vi "Data_get_joe_3.1.vi"() -> ()   [LabVIEW 2011]
uses:
  <vilib>/Utility/error.llb/DialogType.ctl
  <vilib>/Analysis/2dsp.llb/Real FFT.vi
  <vilib>/Analysis/NI_AALPro.lvlib
panel:
  in  "Automatic Overwrite?":bool
  out "f cur. (GHz)":i32
  in  "TDS VISA Port":refnum<visa-resource-name>="GPIB0::1::INSTR"
  in  "Chirp up to (GHz)":dbl
  in  "PauseB":bool caption="Pause"
  in  "Substr":bool
  out "tdsavges#":i32 caption="tds averaged:"
  in  "Auto":bool caption="Autosave"
  in  "FFT every#":u32=1 min=1 max=1000 step=1
  in  "#steps":u32=1 min=1 step=1
  in  "f step (GHz)":dbl=0.0003 min=0.00025 max=67.0 step=1e-06 format="%#.12f"
  in  "time/point":T1(ring)
  in  "time/div":T2(ring)
  out "Current sweep":u32=1 min=1 max=1000 step=1
  in  "Ext":string="ccd"
  in  "Name":string="trace"
  in  "Folder":path
  in  "#Sweeps":u32=1 min=1 max=1000 step=1
  in  "Ampl. (dBm)":dbl min=-135.0 max=30.0 step=0.5 format="%#_8g"
  in  "f start (GHz)":dbl=0.0003 min=0.00025 max=67.0 step=1e-06 format="%#.12f"
  in  "Start":bool
  in  "Quit":bool
  in  "PSG1 VISA Port":refnum<visa-resource-name>="GPIB0::1::INSTR"
  out "read time (ms)":u32
  out "#points":u32
  out "Busy":bool
  in  "Chirp start (MHz)":ext=2.5
  in  "Filter up to (MHz)":ext=2.5
  in  "Amount of averagings":u32=10 min=1 step=1
  out "Data":dbl[](array[numeric])
  out "Frequency Domain Signal":cluster{ext[], dbl[]}(graph)
  out "FFT (Im)":dbl[](array[numeric])
  out "FFT (Re)":dbl[](array[numeric])
  out "Final array":ext[][](array[numeric])
  out "size(s)":i32
  out "Oscilloscope Data":dbl[](array[numeric])
  in  "Channel Number":u16=1
  out "Oscilloscope graph":dbl[](graph)
  in  "Stop":bool
  # "Oscilloscope TDS6124C"
  # "File Storage"
  # "PSG E8257D"
  # "Control"
  # "Spectrum data"
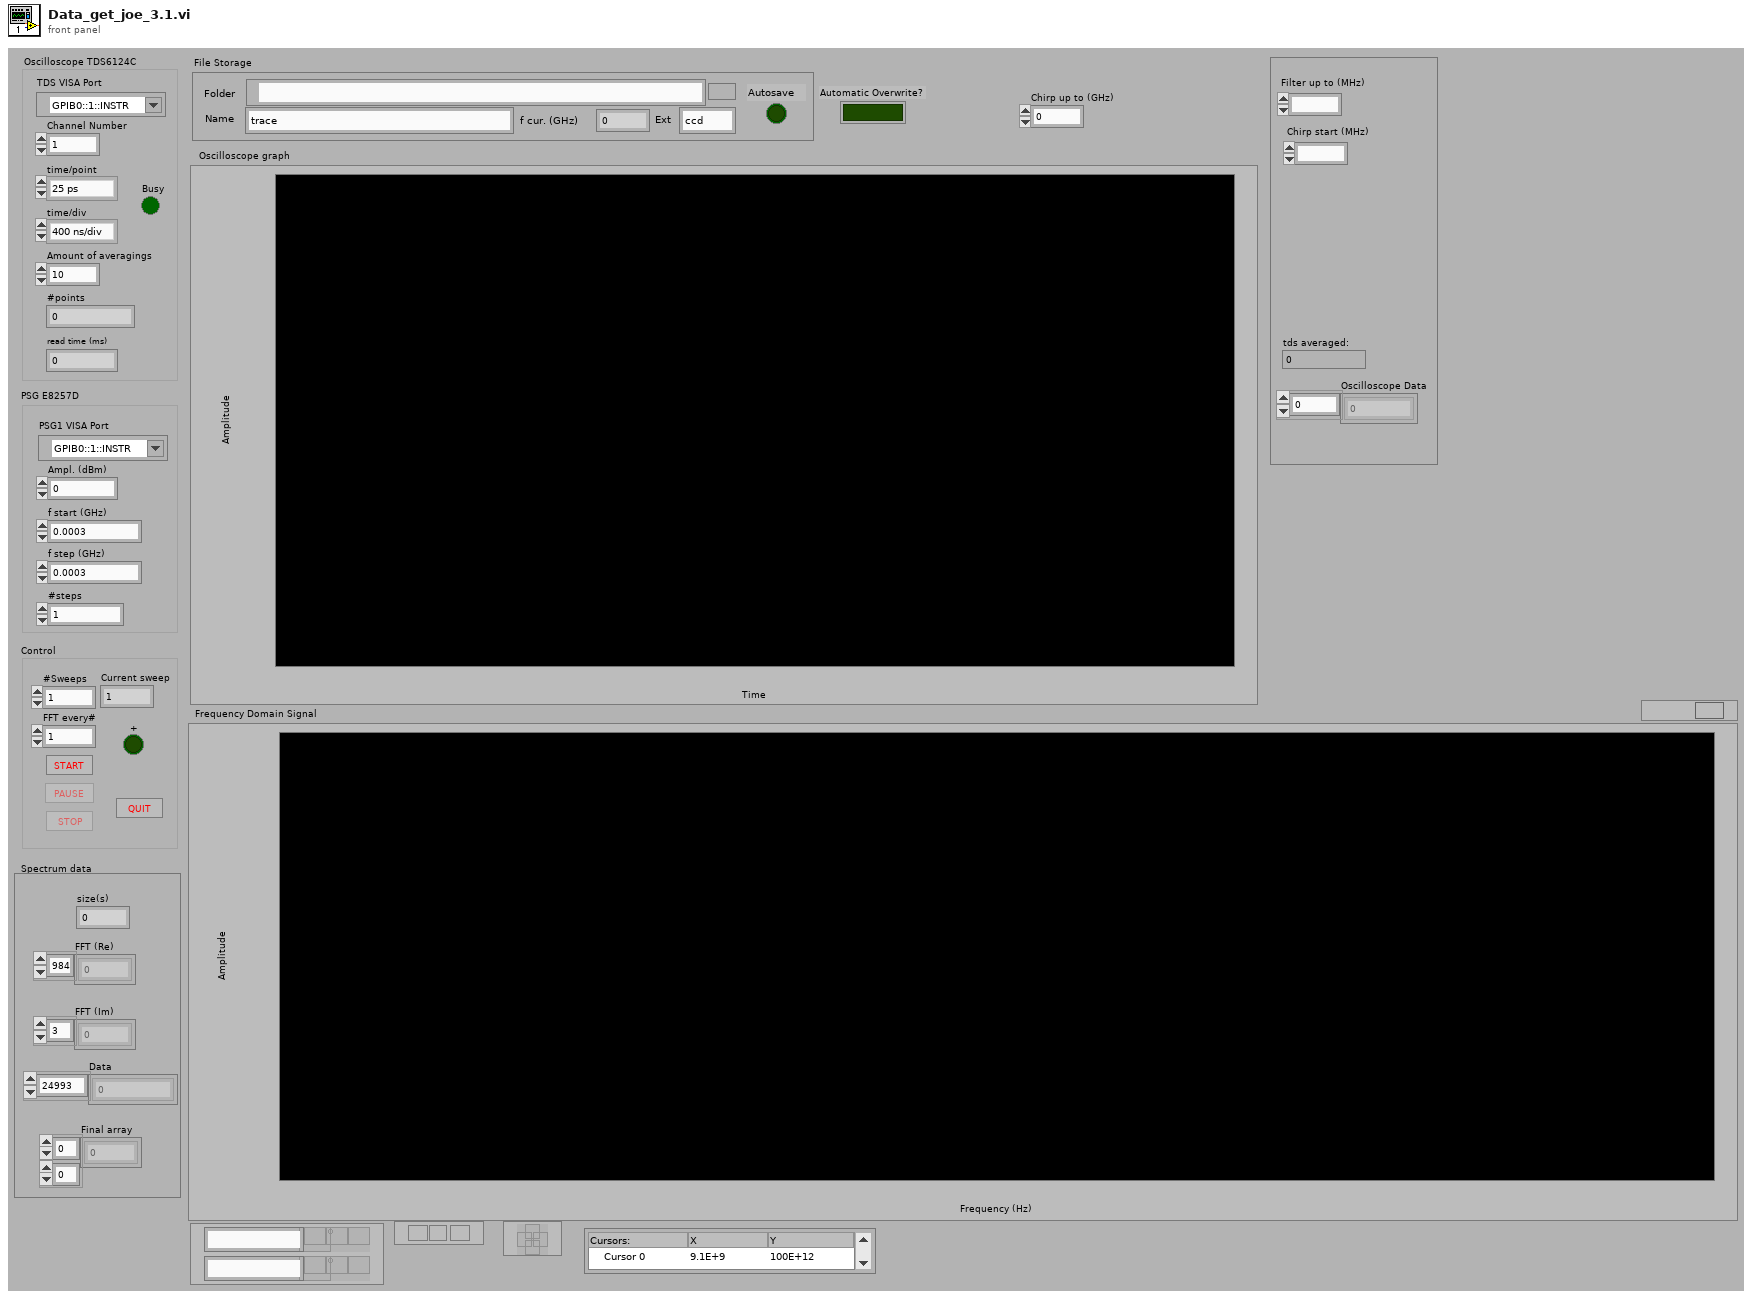
[diagram p1: front panel]
types:
  T1 = enum16{"25 ps", "50 ps", "100 ps", "200 ps", "400 ps", "800 ps", "2 ns"}
  T2 = enum16{"400 ns/div", "1 us/div", "2 us/div", "4 us/div", "10 us/div", "20 us/div"}
  T3 = enum8{"Enabled", "Disabled", "Disabled and Grayed Out"}
  T4 = enum16{"open", "replace", "create", "open or create", "replace or create", "replace or create with confirmation"}
  T5 = typedef "DialogType.ctl" = u16
  T6 = cluster{"Folder":path, "Name":string, "Ext":string}
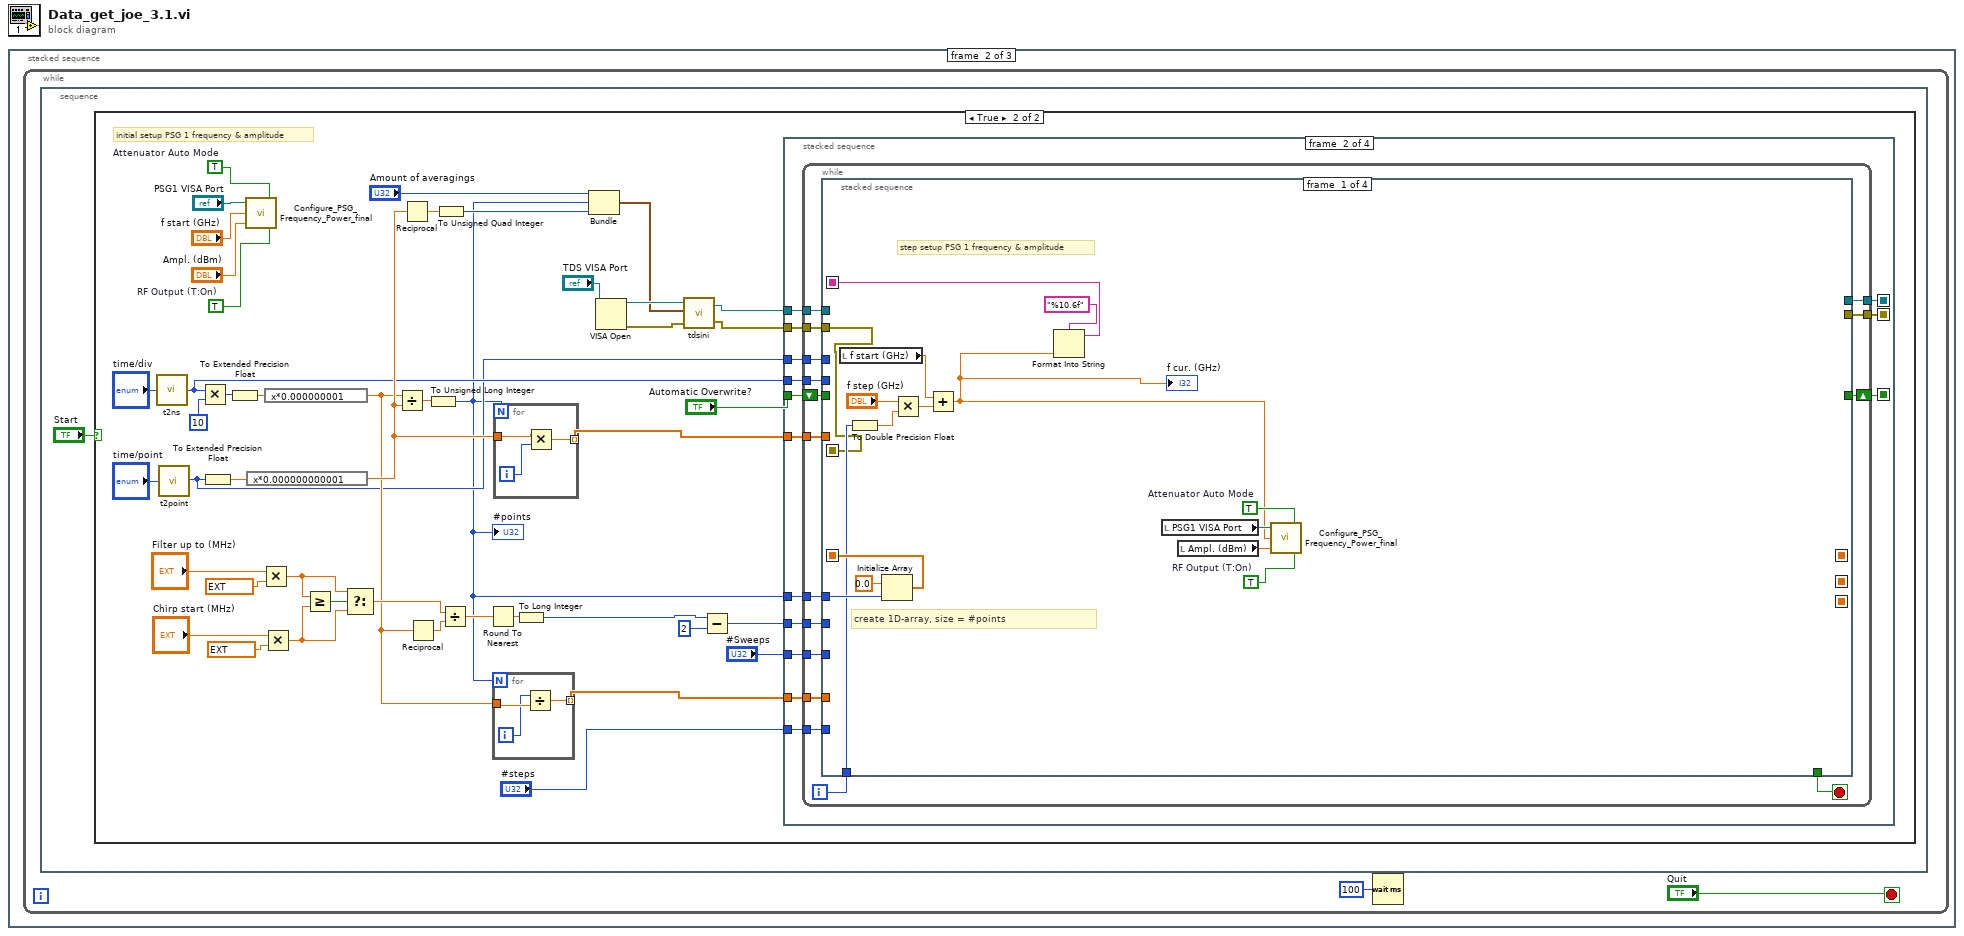
[diagram p0: block diagram]
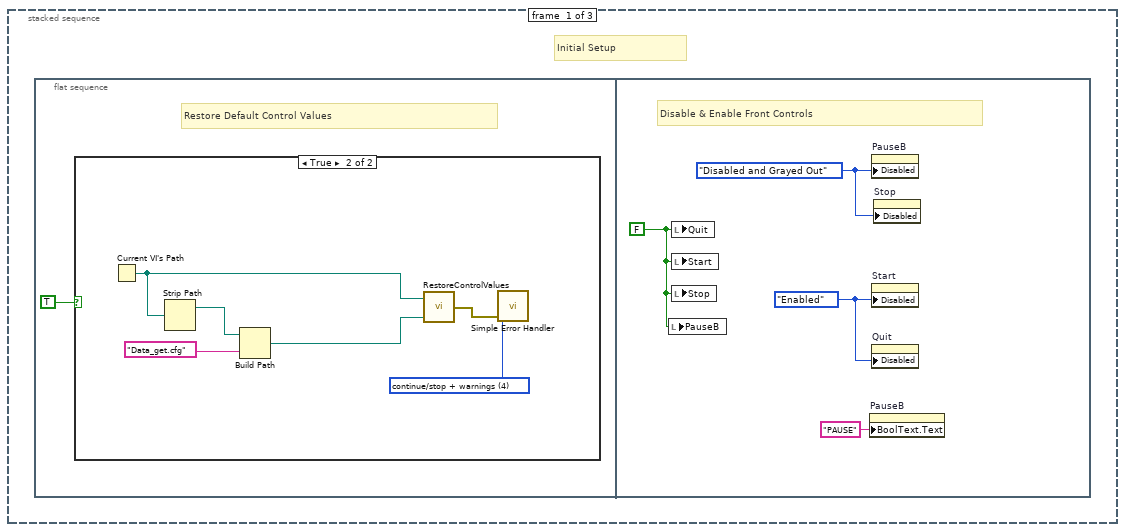
[diagram p2: hidden frame]
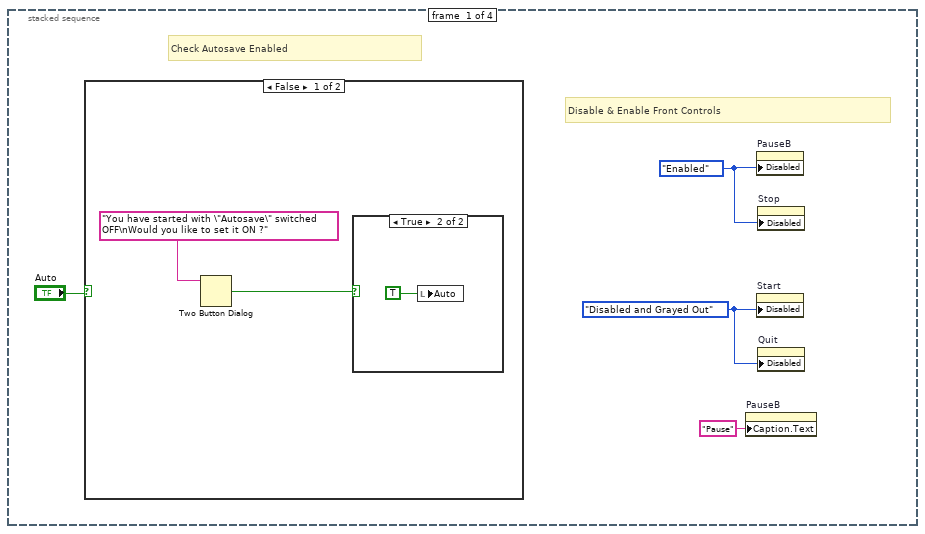
[diagram p5: hidden frame]
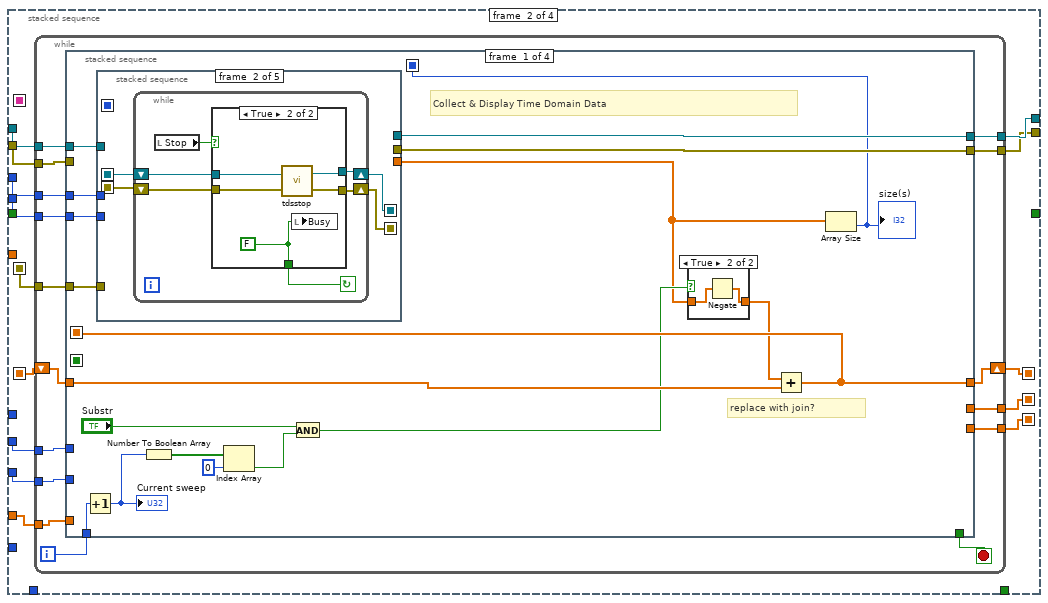
[diagram p8: hidden frame]
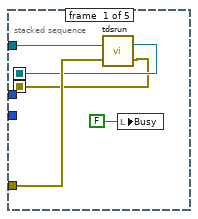
[diagram p10: hidden frame]
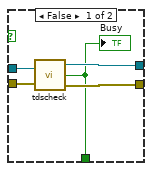
[diagram p11: hidden frame]
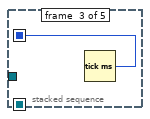
[diagram p12: hidden frame]
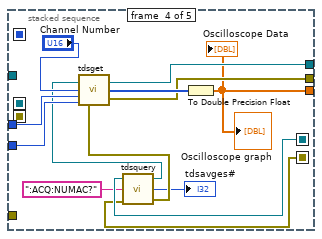
[diagram p13: hidden frame]
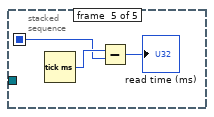
[diagram p14: hidden frame]
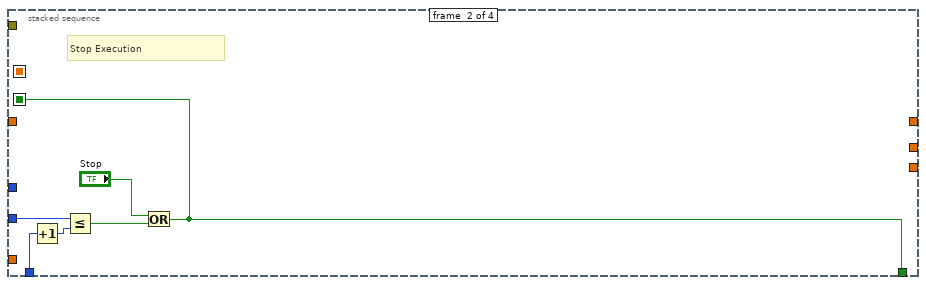
[diagram p15: hidden frame]
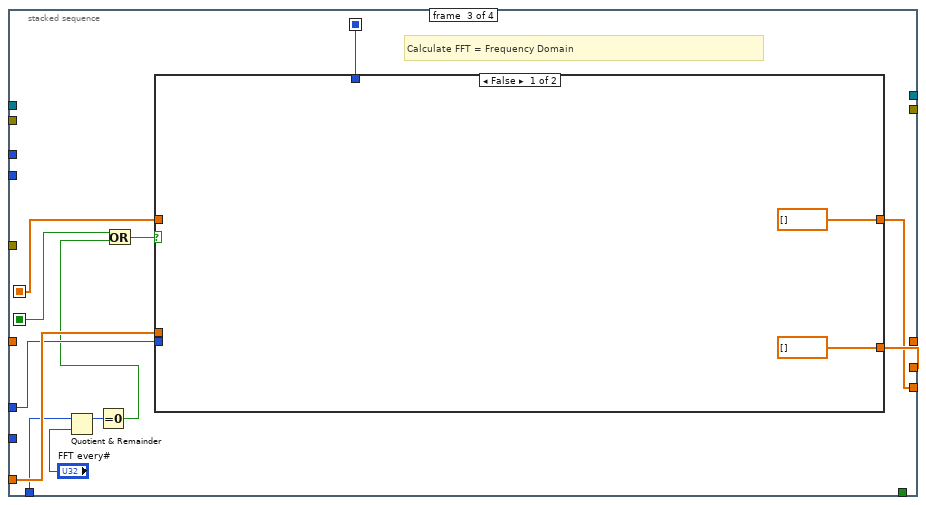
[diagram p16: hidden frame]
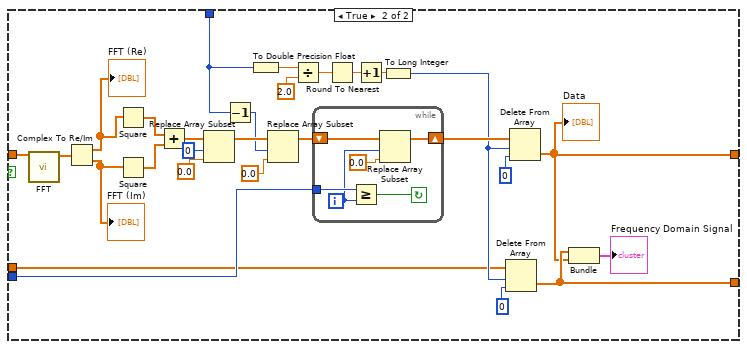
[diagram p17: hidden frame]
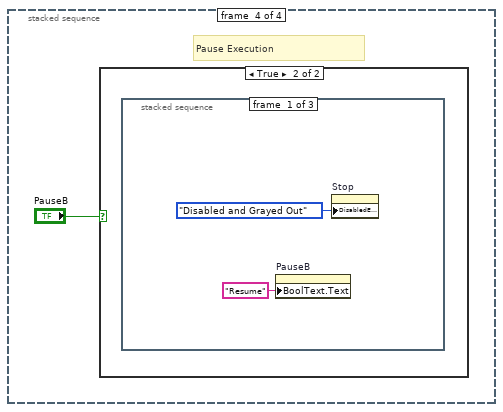
[diagram p18: hidden frame]
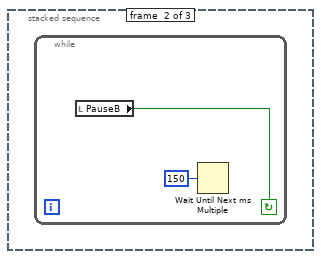
[diagram p20: hidden frame]
diagram:
  n1 = stacked-sequence {
    frame #0 {
      # "Initial Setup"
      n2 = flat-sequence {
        frame #0 {
          # "Restore Default Control Values"
          n3 = case shown="True" TRUE {
            frame False {
            }
            frame True {
              w2 = T5 4 items=["no dialog", "OK message", "continue or stop message", "OK message + warnings", "continue/stop + warnings"] ("type of dialog (OK msg:1)")
              n4 = Current VI's Path() -> (path=w3:path)
              n5 = Strip Path(path=w3) -> (stripped path=w4:path)  [unwired: 1 out]
              n6 = Build Path(base path=w4, name or relative path="Data_get.cfg") -> (appended path=w6:path)
              n7 = call "RestoreControlValues.vi"("file path"=w6, "vi path"=w3) -> ("error out"=w5:errorcluster)
              n8 = call <vilib>:"Simple Error Handler.vi"("type of dialog (OK msg:1)"=w2, "error in (no error)"=w5) -> ()  [unwired: 3 in, 5 out]
            }
          }
        }
        frame #1 {
          w10 = T3."Disabled and Grayed Out" ("Disabled")
          w8 = T3."Enabled" ("Disabled")
          w11 = FALSE ("Quit")
          # "Disable & Enable Front Controls"
          n9 = local write "PauseB"(w11) -> ()
          n10 = local write "Quit"(w11) -> ()
          n11 = local write "Start"(w11) -> ()
          n12 = local write "Stop"(w11) -> ()
          n13 = property on="PauseB" class="Bool (strict)"("BoolText.Text"="PAUSE" ("Boolean Text.Text")) -> ()  [unwired: 2 in, 2 out]
          n14 = property on="PauseB" class="Bool (strict)"("Disabled"=w10) -> ()  [unwired: 2 in, 2 out]
          n15 = property on="Start" class="Bool (strict)"("Disabled"=w8) -> ()  [unwired: 2 in, 2 out]
          n16 = property on="Quit" class="Bool (strict)"("Disabled"=w8) -> ()  [unwired: 2 in, 2 out]
          n17 = property on="Stop" class="Bool (strict)"("Disabled"=w10) -> ()  [unwired: 2 in, 2 out]
        }
      }
    }
    frame #1 {
      n18 = while {
        stop <- "Quit" stop-if-true
        n19 = stacked-sequence {
          frame #0 {
            n20 = case shown="True" "Start" {
              frame False {
              }
              frame True {
                w19 = TRUE  # Attenuator Auto Mode
                w16 = TRUE  # RF Output (T:On)
                # "initial setup PSG 1 frequency & amplitude"
                n21 = call "t2ns.vi"("t/div"="time/div") -> ("ns/div"=w31:u32)
                n22 = call "t2point.vi"("t/point"="time/point") -> ("ps/point"=w29:u32)
                n23 = Multiply(x=w31, y=u32 10) -> (x*y=w54:u32)
                n24 = To Extended Precision Float(1:w29) -> (0:w51:ext)
                n25 = To Extended Precision Float(1:w54) -> (0:w52:ext)
                n26 = call "Configure_PSG_ Frequency_Power_final.vi"("RF Output (T:On)"=w16, "Attenuator Auto Mode (T:Enable)"=w19, "Power [dBm]"="Ampl. (dBm)", "Frequency [GHz]"="f start (GHz)", "VISA resource name"="PSG1 VISA Port") -> ()
                n27 = expression code="x*0.000000000001"(w51) -> (w37:ext)
                n28 = Multiply(x="Filter up to (MHz)", y=ext 1000000.0) -> (x*y=w43:ext)
                n29 = Multiply(x="Chirp start (MHz)", y=ext 1000000.0) -> (x*y=w40:ext)
                n30 = expression code="x*0.000000001"(w52) -> (w33:ext)
                n31 = Greater Or Equal?(x=w43, y=w40) -> (x >= y?=w50:bool)
                n32 = Select(t=w43, s=w50, f=w40) -> (s? t:f=w48:ext)
                n33 = Divide(x=w33, y=w37) -> (x/y=w53:ext)
                n34 = Reciprocal(x=w37) -> (1/x=w35:ext)
                n35 = Reciprocal(x=w33) -> (1/x=w49:ext)
                n36 = To Unsigned Long Integer(number=w53) -> (unsigned 32bit integer=w27:u32)
                "#points" <- w27
                n37 = To Unsigned Quad Integer(1:w35) -> (0:w36:u64)
                n38 = Divide(x=w48, y=w49) -> (x/y=w47:ext)
                n39 = Round To Nearest(number=w47) -> (nearest integer value=w46:ext)
                n40 = for {
                  N: w27 -> [_]
                  tunnel: w33 -> [w458]
                  tunnel: [w459] -> w34 mode=indexing
                  i -> [w457]
                  n41 = Divide(x=w457, y=w458) -> (x/y=w459:ext)
                }
                n42 = for {
                  N: w27 -> [_]
                  tunnel: w37 -> [w462]
                  tunnel: [w461] -> w32 mode=indexing
                  i -> [w460]
                  n43 = Multiply(x=w462, y=w460) -> (x*y=w461:ext)
                }
                n44 = To Long Integer(number=w46) -> (32bit integer=w24:i32)
                n45 = Bundle("Amount of averagings"="Amount of averagings", w27, w36) -> (w38:cluster{"Amount of averagings ":u32, u32, u64})  [unwired: 1 in]
                n46 = VISA Open(VISA resource name="TDS VISA Port") -> (VISA resource name=w56:refnum<visa-resource-name>, error out=w57:errorcluster)  [unwired: 4 in]
                n47 = call "tdsini.vi"("Error In (No Error)"=w57, "Acq_par"=w38, "VISA Port In"=w56) -> ("Error Out"=w58:errorcluster, "VISA Port Out"=w59:refnum<visa-resource-name>)
                n48 = Subtract(x=w24, y=2) -> (x-y=w22:i32)
                n49 = stacked-sequence {
                  seq-local: [_ w73 _ _] -> [_ _ w418 _]
                  seq-local: [_ w72 _ _] -> [_ _ w417 _]
                  seq-local: [_ w67 _ _] -> [_ _ _ w419]
                  tunnel: w59 -> [_ w80 _ _]
                  tunnel: w58 -> [_ w79 _ _]
                  tunnel: w29 -> [_ w78 _ _]
                  tunnel: w31 -> [_ w77 _ _]
                  tunnel: w22 -> [_ w76 _ _]
                  tunnel: w34 -> [_ w75 _ _]
                  tunnel: "#Sweeps" -> [_ w74 _ _]
                  tunnel: w32 -> [_ w69 _ _]
                  tunnel: w27 -> [_ w71 _ _]
                  tunnel: "#steps" -> [_ w70 _ _]
                  tunnel: "Automatic Overwrite?" -> [_ w68 _ _]
                  frame #0 {
                    w61 = T3."Enabled" ("Disabled")
                    w60 = T3."Disabled and Grayed Out" ("Disabled")
                    # "Check Autosave Enabled"
                    # "Disable & Enable Front Controls"
                    n50 = case shown="False" "Auto" {
                      frame False {
                        n51 = Two Button Dialog(message="You have started with \"Autosave\" switched OFF\nWould you like to set it ON ?") -> (T button?=w64:bool)  [unwired: 2 in]
                        n52 = case shown="True" w64 {
                          frame False {
                          }
                          frame True {
                            n53 = local write "Auto"(TRUE) -> ()
                          }
                        }
                      }
                      frame True {
                      }
                    }
                    n54 = property on="PauseB" class="Bool (strict)"("Caption.Text"="Pause") -> ()  [unwired: 2 in, 2 out]
                    n55 = property on="PauseB" class="Bool (strict)"("Disabled"=w61) -> ()  [unwired: 2 in, 2 out]
                    n56 = property on="Start" class="Bool (strict)"("Disabled"=w60) -> ()  [unwired: 2 in, 2 out]
                    n57 = property on="Stop" class="Bool (strict)"("Disabled"=w61) -> ()  [unwired: 2 in, 2 out]
                    n58 = property on="Quit" class="Bool (strict)"("Disabled"=w60) -> ()  [unwired: 2 in, 2 out]
                  }
                  frame #1 {
                    n59 = while {
                      tunnel: w80 -> [w96]
                      tunnel: w79 -> [w95]
                      tunnel: w78 -> [w94]
                      tunnel: w77 -> [w93]
                      tunnel: w76 -> [w92]
                      tunnel: w75 -> [w91]
                      tunnel: w74 -> [w90]
                      tunnel: [w89] -> w73
                      tunnel: [w88] -> w72
                      tunnel: w71 -> [w87]
                      tunnel: w70 -> [w85]
                      tunnel: w69 -> [w83]
                      shift-right: [w81] -> w67
                      shift-left: w68 -> [w82]
                      i -> [w86]
                      stop <- w84 stop-if-true
                      n60 = stacked-sequence {
                        seq-local: [w111 _ _ _] -> [_ w117 _ _]
                        seq-local: [w102 _ _ _] -> [_ w116 _ _]
                        seq-local: [_ w115 _ _] -> [_ _ w273 _]
                        seq-local: [_ w114 _ _] -> [_ _ w272 _]
                        seq-local: [_ w113 _ _] -> [_ _ w271 _]
                        seq-local: [w103 _ _ _] -> [_ _ w270 _]
                        tunnel: w96 -> [_ w126 _ _]
                        tunnel: w95 -> [w102 w125 _ _]
                        tunnel: w94 -> [_ w124 _ _]
                        tunnel: w93 -> [_ w123 _ _]
                        tunnel: w92 -> [_ w122 _ _]
                        tunnel: w91 -> [_ w121 _ _]
                        tunnel: w90 -> [_ w120 _ _]
                        tunnel: [_ w119 _ _] -> w89
                        tunnel: [_ w118 _ _] -> w88
                        tunnel: w87 -> [w110 _ _ _]
                        tunnel: w86 -> [w107 _ _ w411]
                        tunnel: w85 -> [_ _ _ w410]
                        tunnel: [_ _ _ w409] -> w84
                        tunnel: w83 -> [_ _ w274 _]
                        tunnel: w82 -> [_ _ w268 _]
                        tunnel: [_ _ w267 _] -> w81
                        frame #0 {
                          w101 = TRUE  # Attenuator Auto Mode
                          w100 = TRUE  # RF Output (T:On)
                          # "step setup PSG 1 frequency & amplitude"
                          # "create 1D-array, size = #points"
                          n61 = local read "f start (GHz)"() -> (w105:dbl)
                          n62 = To Double Precision Float(number=w107) -> (double precision float=w108:dbl)
                          n63 = Initialize Array(0.0 ("element"), w110) -> (w111:dbl[])
                          n64 = Multiply(x="f step (GHz)", y=w108) -> (x*y=w106:dbl)
                          n65 = Add(x=w105, y=w106) -> (x+y=w98:dbl)
                          "f cur. (GHz)" <- w98
                          n66 = Format Into String(format string="%10.6f", w98) -> (resulting string=w103:string)  [unwired: 2 in, 1 out]
                          n67 = local read "PSG1 VISA Port"() -> (w99:refnum<visa-resource-name>)
                          n68 = local read "Ampl. (dBm)"() -> (w97:dbl)
                          n69 = call "Configure_PSG_ Frequency_Power_final.vi"("RF Output (T:On)"=w100, "Attenuator Auto Mode (T:Enable)"=w101, "Power [dBm]"=w97, "Frequency [GHz]"=w98, "VISA resource name"=w99) -> ()
                        }
                        frame #1 {
                          n70 = while {
                            tunnel: [w139] -> w118
                            tunnel: [w140] -> w119
                            tunnel: w125 -> [w141]
                            tunnel: w126 -> [w142]
                            tunnel: w124 -> [w138]
                            tunnel: w123 -> [w137]
                            tunnel: w121 -> [w135]
                            tunnel: w122 -> [w136]
                            tunnel: w120 -> [w132]
                            shift-right: [w130] -> w115
                            shift-left: w117 -> [w131]
                            tunnel: [w129] -> w114
                            tunnel: w116 -> [w128]
                            tunnel: [w127] -> w113
                            i -> [w134]
                            stop <- w133 stop-if-true
                            n71 = stacked-sequence {
                              seq-local: [w152 _ _ _] -> [_ _ w223 _]
                              seq-local: [w153 _ _ _] -> [_ _ w222 _]
                              seq-local: [_ w206 _ _] -> [_ _ w213 _]
                              tunnel: w142 -> [w160 _ _ _]
                              tunnel: w141 -> [_ _ _ _]
                              tunnel: [w159 _ _ _] -> w140
                              tunnel: [w158 _ _ _] -> w139
                              tunnel: w138 -> [w157 _ _ _]
                              tunnel: w137 -> [w156 _ _ _]
                              tunnel: w136 -> [_ _ w220 _]
                              tunnel: w135 -> [_ _ w221 _]
                              tunnel: w134 -> [w151 w211 w217 _]
                              tunnel: [_ w206 _ _] -> w133
                              tunnel: w132 -> [_ w208 _ _]
                              tunnel: w131 -> [w155 _ _ _]
                              tunnel: [w153 _ _ _] -> w130
                              tunnel: [_ _ w219 _] -> w129
                              tunnel: w128 -> [w154 _ _ _]
                              tunnel: [_ _ w218 _] -> w127
                              frame #0 {
                                # "replace with join?"
                                # "Collect & Display Time Domain Data"
                                n72 = Increment(x=w151) -> (x+1=w143:i32)
                                "Current sweep" <- w143
                                n73 = stacked-sequence {
                                seq-local: [w166 _ _ _ _] -> [_ w172 _ _ _]
                                seq-local: [w165 _ _ _ _] -> [_ w171 _ _ _]
                                seq-local: [_ w169 _ _ _] -> [_ _ _ w194 _]
                                seq-local: [_ w170 _ _ _] -> [_ _ _ w195 _]
                                seq-local: [_ _ w189 _ _] -> [_ _ _ _ w204]
                                tunnel: w160 -> [w167 _ _ _ _]
                                tunnel: w154 -> [w168 _ _ _ _]
                                tunnel: [_ _ _ w201 _] -> w159
                                tunnel: [_ _ _ w200 _] -> w158
                                tunnel: w157 -> [_ _ _ w198 _]
                                tunnel: w156 -> [_ _ _ w197 _]
                                tunnel: [_ _ _ w196 _] -> w146
                                frame #0 {
                                n74 = call "tdsrun.vi"("Error In (No Error)"=w168, "VISA Port In"=w167) -> ("Error Out"=w165:errorcluster, "VISA Port Out"=w166:refnum<visa-resource-name>)
                                n75 = local write "Busy"(FALSE ("Busy")) -> ()
                                }
                                frame #1 {
                                n76 = while {
                                shift-right: [w176] -> w170
                                shift-left: w172 -> [w177]
                                shift-right: [w175] -> w169
                                shift-left: w171 -> [w178]
                                stop <- w174 continue-if-true
                                n77 = local read "Stop"() -> (w173:bool)
                                n78 = case shown="True" w173 {
                                tunnel: w178 -> [w183 w187]
                                tunnel: w177 -> [w182 w188]
                                tunnel: [w181 w185] -> w176
                                tunnel: [w180 w186] -> w175
                                tunnel: [w179 w184] -> w174
                                frame False {
                                n79 = call "tdscheck.vi"("VISA Port In"=w182, "Error In (No Error)"=w183) -> ("VISA Port Out"=w181:refnum<visa-resource-name>, "busy"=w179:bool, "Error Out"=w180:errorcluster)
                                "Busy" <- w179
                                }
                                frame True {
                                w184 = FALSE ("busy")
                                n80 = call "tdsstop.vi"("Error In (No Error)"=w187, "VISA Port In"=w188) -> ("Error Out"=w186:errorcluster, "VISA Port Out"=w185:refnum<visa-resource-name>)
                                n81 = local write "Busy"(w184) -> ()
                                }
                                }
                                }
                                }
                                frame #2 {
                                n82 = Tick Count (ms)() -> (millisecond timer value=w189:u32)
                                }
                                frame #3 {
                                n83 = call "tdsquery.vi"("Error In (No Error)"=w194, "String to TDS"=":ACQ:NUMAC?", "VISA Port In"=w195) -> ("Error Out"=w191:errorcluster, "number"=→"tdsavges#":i32, "VISA Port Out"=w192:refnum<visa-resource-name>)
                                n84 = call "tdsget.vi"("VISA Port In"=w192, "Channel Number"="Channel Number", "ps/point"=w198, "ns/div"=w197, "Error In (No Error)"=w191) -> ("VISA Port Out"=w201:refnum<visa-resource-name>, "TDS Data"=w202:u16[], "Error Out"=w200:errorcluster)  [unwired: 8 in]
                                n85 = To Double Precision Float(number=w202) -> (double precision float=w196:dbl[])
                                "Oscilloscope graph" <- w196
                                "Oscilloscope Data" <- w196
                                }
                                frame #4 {
                                n86 = Tick Count (ms)() -> (millisecond timer value=w205:u32)
                                n87 = Subtract(x=w205, y=w204) -> (x-y=→"read time (ms)":u32)
                                }
                                }
                                n88 = Number To Boolean Array(number=w143) -> (Boolean array=w150:bool[])
                                n89 = Index Array(array=w150, index=0) -> (element=w148:bool)
                                n90 = And(x="Substr", y=w148) -> (x .and. y?=w147:bool)
                                n91 = case shown="True" w147 {
                                tunnel: w146 -> [w161 w163]
                                tunnel: [w161 w162] -> w145
                                frame False {
                                }
                                frame True {
                                n92 = Negate(x=w163) -> (-x=w162:dbl[])
                                }
                                }
                                n93 = Add(x=w145, y=w155) -> (x+y=w153:dbl[])
                                n94 = Array Size(array=w146) -> (size(s)=w152:i32)
                                "size(s)" <- w152
                              }
                              frame #1 {
                                # "Stop Execution"
                                n95 = Increment(x=w211) -> (x+1=w207:i32)
                                n96 = Less Or Equal?(x=w208, y=w207) -> (x <= y?=w210:bool)
                                n97 = Or(x="Stop", y=w210) -> (x .or. y?=w206:bool)
                              }
                              frame #2 {
                                # "Calculate FFT = Frequency Domain"
                                n98 = Quotient & Remainder(x=w217, y="FFT every#") -> (x-y*floor(x/y)=w215:u32)  [unwired: 1 out]
                                n99 = Equal To 0?(x=w215) -> (x = 0?=w212:bool)
                                n100 = Or(x=w213, y=w212) -> (x .or. y?=w214:bool)
                                n101 = case shown="False" w214 {
                                tunnel: w223 -> [_ w231]
                                tunnel: w222 -> [_ w230]
                                tunnel: w221 -> [_ w226]
                                tunnel: w220 -> [_ w229]
                                tunnel: [ext[] [] w228] -> w219
                                tunnel: [dbl[] [] w227] -> w218
                                frame False {
                                }
                                frame True {
                                n102 = call-poly <vilib>:"FFT.vi"("X"=w230) -> ("FFT {X}"=w253:cdb[])  [unwired: 9 in, 1 out]
                                n103 = Complex To Re/Im(x + iy=w253) -> (x=w252:dbl[], y=w251:dbl[])
                                "FFT (Re)" <- w252
                                "FFT (Im)" <- w251
                                n104 = Square(x=w252) -> (x^2=w250:dbl[])
                                n105 = Square(x=w251) -> (x^2=w249:dbl[])
                                n106 = Add(x=w250, y=w249) -> (x+y=w245:dbl[])
                                n107 = Replace Array Subset(array=w245, new element=0.0 ("new element/subarray"), index=0) -> (w244:dbl[])
                                n108 = Decrement(x=w231) -> (x-1=w243:i32)
                                n109 = To Double Precision Float(number=w231) -> (double precision float=w239:dbl)
                                n110 = Replace Array Subset(array=w244, new element=0.0 ("new element/subarray"), index=w243) -> (w241:dbl[])
                                n111 = Divide(x=w239, y=2.0) -> (x/y=w237:dbl)
                                n112 = while {
                                tunnel: w229 -> [w258]
                                shift-right: [w256] -> w240
                                shift-left: w241 -> [w257]
                                i -> [w255]
                                stop <- w259 continue-if-true
                                n113 = Greater Or Equal?(x=w258, y=w255) -> (x >= y?=w259:bool)
                                n114 = Replace Array Subset(array=w257, new element=0.0 ("new element/subarray"), index=w255) -> (w256:dbl[])
                                }
                                n115 = Round To Nearest(number=w237) -> (nearest integer value=w236:dbl)
                                n116 = Increment(x=w236) -> (x+1=w235:dbl)
                                n117 = To Long Integer(number=w235) -> (32bit integer=w232:i32)
                                n118 = Delete From Array(array=w226, length=w232, index=0) -> (deleted portion=w228:ext[])  [unwired: 1 out]
                                n119 = Delete From Array(array=w240, length=w232, index=0) -> (deleted portion=w227:dbl[])  [unwired: 1 out]
                                "Data" <- w227
                                n120 = Bundle(w228, w227) -> (→"Frequency Domain Signal":cluster{ext[], dbl[]})  [unwired: 1 in]
                                }
                                }
                              }
                              frame #3 {
                                # "Pause Execution"
                                n121 = case shown="True" "PauseB" {
                                frame False {
                                }
                                frame True {
                                n122 = stacked-sequence {
                                frame #0 {
                                n123 = property on="PauseB" class="Bool (strict)"("BoolText.Text"="Resume" ("Caption.Text")) -> ()  [unwired: 2 in, 2 out]
                                n124 = property on="Stop" class="Bool (strict)"("DisabledEnum"=T3."Disabled and Grayed Out" ("Disabled")) -> ()  [unwired: 2 in, 2 out]
                                }
                                frame #1 {
                                n125 = while {
                                stop <- w264 continue-if-true
                                n126 = local read "PauseB"() -> (w264:bool)
                                n127 = Wait Until Next ms Multiple(millisecond multiple=u32 150) -> ()  [unwired: 1 out]
                                }
                                }
                                frame #2 {
                                n128 = property on="PauseB" class="Bool (strict)"("BoolText.Text"="Pause" ("Caption.Text")) -> ()  [unwired: 2 in, 2 out]
                                n129 = property on="Stop" class="Bool (strict)"("DisabledEnum"=T3."Enabled" ("Disabled")) -> ()  [unwired: 2 in, 2 out]
                                }
                                }
                                }
                                }
                              }
                            }
                          }
                        }
                        frame #2 {
                          # "Auto Safe?"
                          n130 = local read "Auto"() -> (w269:bool)
                          n131 = case shown="True" w269 {
                            tunnel: w274 -> [_ w282]
                            tunnel: w273 -> [_ w281]
                            tunnel: w272 -> [_ w280]
                            tunnel: w271 -> [_ w279]
                            tunnel: w270 -> [_ w278]
                            tunnel: w268 -> [_ w277]
                            tunnel: [FALSE w276] -> w267
                            frame False {
                            }
                            frame True {
                              n132 = stacked-sequence {
                                seq-local: [w283 _ _ _] -> [_ w307 _ _]
                                seq-local: [_ _ w361 _] -> [_ _ _ w401]
                                seq-local: [_ w293 _ _] -> [_ _ _ w392]
                                tunnel: w282 -> [_ w309 _ _]
                                tunnel: w281 -> [_ w296 _ _]
                                tunnel: w280 -> [_ _ _ w404]
                                tunnel: w279 -> [_ _ _ w403]
                                tunnel: w278 -> [w286 w295 w363 _]
                                tunnel: w277 -> [_ w299 _ _]
                                tunnel: [_ w293 _ _] -> w276
                                frame #0 {
                                # "create complete filename incl. path as a string"
                                n133 = Path To String(path="Folder") -> (string=w291:string)
                                n134 = Concatenate Strings(w291, "\\\\" ("string"), "Name", "_", "td", w286, ".", "Ext") -> (w283:string)
                                }
                                frame #1 {
                                # "(%e) = Scientific Notation"
                                n135 = Build Array(w309, w296) -> (w311:ext[][])
                                n136 = String To Path(string=w307) -> (path=w298:path)
                                n137 = case shown="False" w299 {
                                tunnel: w307 -> [w313 _]
                                tunnel: [w318 w359] -> w293
                                tunnel: [w316 T4."replace or create" ("operation (0:open)")] -> w301
                                tunnel: w299 -> [w317 w359]
                                tunnel: w298 -> [w315 w358]
                                tunnel: [w314 w358] -> w297
                                tunnel: w295 -> [w312 _]
                                frame False {
                                n138 = call "CheckFileExist.vi"("Path"=w313) -> ("File Exists"=w320:bool, "Overwrite File"=w319:bool)  [unwired: 1 in, 1 out]
                                n139 = case "check file existance" shown="True" w320 {
                                tunnel: w319 -> [_ w329]
                                tunnel: [w323 w327] -> w318
                                tunnel: w317 -> [w323 _]
                                tunnel: [T4."create" ("operation (0:open)") w328] -> w316
                                tunnel: w315 -> [w321 w326]
                                tunnel: [w321 w325] -> w314
                                tunnel: w312 -> [_ w324]
                                frame False {
                                # "file doesn't exist"
                                }
                                frame True {
                                # "file exists"
                                n140 = case shown="False" w329 {
                                tunnel: [w332 T4."replace or create" ("operation (0:open)")] -> w328
                                tunnel: [w333 TRUE] -> w327
                                tunnel: w326 -> [_ w355]
                                tunnel: [w330 w355] -> w325
                                tunnel: w324 -> [w331 _]
                                frame False {
                                # "file exists and should not be overwritten"
                                n141 = stacked-sequence {
                                tunnel: [_ _ FALSE] -> w333
                                tunnel: [_ _ T4."create" ("operation (0:open)")] -> w332
                                tunnel: w331 -> [_ w342 _]
                                tunnel: [_ w347 _] -> w330
                                frame #0 {
                                # "enter new file name"
                                n142 = local read "Folder"() -> (w341:path)
                                n143 = local read "Name"() -> (w340:string)
                                n144 = local read "Ext"() -> (w339:string)
                                n145 = Bundle("Folder"=w341, "Name"=w340, "Ext"=w339) -> (w338:T6)  [unwired: 1 in]
                                n146 = call "ChangeFileName.vi"("input par"=w338) -> ("output par"=w337:T6)  [unwired: 1 out]
                                n147 = Unbundle(w337) -> ("Folder"=w336:path, "Name"=w335:string, "Ext"=w334:string)
                                n148 = local write "Folder"(w336) -> ()
                                n149 = local write "Name"(w335) -> ()
                                n150 = local write "Ext"(w334) -> ()
                                }
                                frame #1 {
                                # "create new path"
                                n151 = local read "Ext"() -> (w344:string)
                                n152 = local read "Folder"() -> (w349:path)
                                n153 = local read "Name"() -> (w348:string)
                                n154 = Path To String(path=w349) -> (string=w352:string)
                                n155 = Concatenate Strings(w352, "\\\\" ("string"), w348, "_", "td", w342, ".", w344) -> (w343:string)
                                n156 = String To Path(string=w343) -> (path=w347:path)
                                }
                                frame #2 {
                                }
                                }
                                }
                                frame True {
                                # "overwrite existing file"
                                }
                                }
                                }
                                }
                                }
                                frame True {
                                }
                                }
                                n157 = Transpose 2D Array(2D array=w311) -> (transposed array=w308:ext[][])
                                n158 = Array To Spreadsheet String(array=w308, 3:"%e") -> (spreadsheet string=w300:string)  [unwired: 1 in]
                                n159 = Open/Create/Replace File(file path (use dialog)=w297, operation (0:open)=w301, access (0:read/write)=enum16{"read/write", "read-only", "write-only"}."write-only") -> (refnum out=w303:refnum<file>, error out=w306:errorcluster)  [unwired: 3 in, 1 out]
                                n160 = Write to Text File(file (use dialog)=w303, text=w300, error in=w306) -> (refnum out=w304:refnum<file>, error out=w305:errorcluster)  [unwired: 1 in, 1 out]
                                n161 = Close File(refnum=w304, error in=w305) -> (error out=w294:errorcluster)  [unwired: 1 out]
                                n162 = call <vilib>:"Simple Error Handler.vi"("error in (no error)"=w294) -> ()  [unwired: 4 in, 5 out]
                                }
                                frame #2 {
                                n163 = local read "Folder"() -> (w365:path)
                                n164 = local read "Name"() -> (w364:string)
                                n165 = local read "Ext"() -> (w362:string)
                                n166 = Path To String(path=w365) -> (string=w371:string)
                                n167 = Concatenate Strings(w371, "\\\\" ("string"), w364, "_") -> (w366:string)
                                n168 = Concatenate Strings(w366, "sd", w363, ".", w362) -> (w361:string)
                                }
                                frame #3 {
                                n169 = Multiply(x="Chirp up to (GHz)", y=1000000000.0) -> (x*y=w373:dbl)
                                n170 = To Extended Precision Float(1:w373) -> (0:w372:ext)
                                n171 = To Extended Precision Float(1:w403) -> (0:w405:ext[])
                                n172 = Build Array(w404, w405) -> (w402:ext[][])
                                n173 = String To Path(string=w401) -> (path=w394:path)
                                n174 = case shown="True" w392 {
                                tunnel: [T4."replace or create with confirmation" ("operation (0:open)") T4."replace or create" ("operation (0:open)")] -> w393
                                frame False {
                                }
                                frame True {
                                }
                                }
                                n175 = Transpose 2D Array(2D array=w402) -> (transposed array=w375:ext[][])
                                n176 = Index Array(array=w375, index (col)=0 ("disabled index (col)")) -> (element=w385:ext[])  [unwired: 1 in]
                                n177 = Index Array(array=w385, index=1) -> (element=w387:ext)
                                n178 = Index Array(array=w385, index=0) -> (element=w386:ext)
                                n179 = Subtract(x=w387, y=w386) -> (x-y=w382:ext)
                                n180 = Divide(x=w372, y=w382) -> (x/y=w379:ext)
                                n181 = Round To Nearest(number=w379) -> (nearest integer value=w381:ext)
                                n182 = To Long Integer(number=w381) -> (32bit integer=w380:i32)
                                n183 = Increment(x=w380) -> (x+1=w376:i32)
                                n184 = Array Subset(array=w375, index (row)=0 ("index"), length (row)=w376, index (col)=0 ("index"), length (col)=w376) -> (w374:ext[][])
                                "Final array" <- w374
                                n185 = Array To Spreadsheet String(array=w374, 3:"%e") -> (spreadsheet string=w395:string)  [unwired: 1 in]
                                n186 = Open/Create/Replace File(file path (use dialog)=w394, operation (0:open)=w393, access (0:read/write)=enum16{"read/write", "read-only", "write-only"}."write-only") -> (refnum out=w397:refnum<file>, error out=w400:errorcluster)  [unwired: 3 in, 1 out]
                                n187 = Write to Text File(file (use dialog)=w397, text=w395, error in=w400) -> (refnum out=w398:refnum<file>, error out=w399:errorcluster)  [unwired: 1 in, 1 out]
                                n188 = Close File(refnum=w398, error in=w399) -> (error out=w391:errorcluster)  [unwired: 1 out]
                                n189 = call <vilib>:"Simple Error Handler.vi"("error in (no error)"=w391) -> ()  [unwired: 4 in, 5 out]
                                }
                              }
                            }
                          }
                        }
                        frame #3 {
                          n190 = Increment(x=w411) -> (x+1=w413:i32)
                          n191 = Less Or Equal?(x=w410, y=w413) -> (x <= y?=w414:bool)
                          n192 = local read "Stop"() -> (w412:bool)
                          n193 = Or(x=w412, y=w414) -> (x .or. y?=w409:bool)
                        }
                      }
                    }
                  }
                  frame #2 {
                    w416 = T3."Disabled and Grayed Out" ("Disabled")
                    w415 = T3."Enabled" ("Disabled")
                    n194 = property on="Quit" class="Bool (strict)"("Disabled"=w415) -> ()  [unwired: 2 in, 2 out]
                    n195 = property on="PauseB" class="Bool (strict)"("Disabled"=w416) -> ()  [unwired: 2 in, 2 out]
                    n196 = property on="Stop" class="Bool (strict)"("Disabled"=w416) -> ()  [unwired: 2 in, 2 out]
                    n197 = property on="Start" class="Bool (strict)"("Disabled"=w415) -> ()  [unwired: 2 in, 2 out]
                    n198 = VISA Close(VISA resource name=w418, error in (no error)=w417) -> ()  [unwired: 1 out]
                  }
                  frame #3 {
                    n199 = local read "Auto"() -> (w420:bool)
                    n200 = case shown="True" w420 {
                      tunnel: w419 -> [_ w423]
                      frame False {
                      }
                      frame True {
                        # "safe measurement settings to file"
                        n201 = local read "time/point"() -> (w452:T1)
                        n202 = local read "time/div"() -> (w451:T2)
                        n203 = local read "Channel Number"() -> (w453:u16)
                        n204 = local read "Amount of averagings"() -> (w450:u32)
                        n205 = local read "#Sweeps"() -> (w449:u32)
                        n206 = local read "Filter up to (MHz)"() -> (w448:ext)
                        n207 = local read "Chirp start (MHz)"() -> (w447:ext)
                        n208 = local read "Ampl. (dBm)"() -> (w446:dbl)
                        n209 = local read "f start (GHz)"() -> (w443:dbl)
                        n210 = local read "f step (GHz)"() -> (w442:dbl)
                        n211 = local read "#steps"() -> (w441:u32)
                        n212 = call "t2point.vi"("t/point"=w452) -> ("ps/point"=w444:u32)
                        n213 = call "t2ns.vi"("t/div"=w451) -> ("ns/div"=w445:u32)
                        n214 = local read "Folder"() -> (w437:path)
                        n215 = local read "Name"() -> (w436:string)
                        n216 = local read "Ext"() -> (w433:string)
                        n217 = Path To String(path=w437) -> (string=w440:string)
                        n218 = Format Into String(format string="Channel: %d\\nps/point: %d\\nns/div: %d\\nAmount of averagings: %d\\n#Sweeps: %d\\nFilter up to (MHz): %f\\nChirp start (MHz): %f\\nAmpl. (dBm): %f\\nf start (GHz): %f\\nf step (MHz): %f\\n#steps: %d\\n", w453, w444, w445, w450, w449, w448, w447, w446, w443, w442, w441) -> (resulting string=w424:string)  [unwired: 2 in, 1 out]
                        n219 = case shown="True" w423 {
                          tunnel: [T4."replace or create with confirmation" ("operation (0:open)") T4."replace or create" ("operation (0:open)")] -> w422
                          frame False {
                          }
                          frame True {
                          }
                        }
                        n220 = Concatenate Strings(w440, "\\\\" ("string"), w436, "_", "par", ".", w433) -> (w432:string)
                        n221 = String To Path(string=w432) -> (path=w426:path)
                        n222 = Open/Create/Replace File(file path (use dialog)=w426, operation (0:open)=w422, access (0:read/write)=enum16{"read/write", "read-only", "write-only"}."write-only") -> (refnum out=w428:refnum<file>, error out=w431:errorcluster)  [unwired: 3 in, 1 out]
                        n223 = Write to Text File(file (use dialog)=w428, text=w424, error in=w431) -> (refnum out=w429:refnum<file>, error out=w430:errorcluster)  [unwired: 1 in, 1 out]
                        n224 = Close File(refnum=w429, error in=w430) -> (error out=w427:errorcluster)  [unwired: 1 out]
                        n225 = call <vilib>:"Simple Error Handler.vi"("error in (no error)"=w427) -> ()  [unwired: 4 in, 5 out]
                      }
                    }
                    n226 = local write "Stop"(FALSE ("Stop")) -> ()
                  }
                }
              }
            }
          }
        }
        n227 = Wait (ms)(milliseconds to wait=u32 100) -> ()  [unwired: 1 out]
      }
    }
    frame #2 {
      n228 = Current VI's Path() -> (path=w463:path)
      n229 = Strip Path(path=w463) -> (stripped path=w464:path)  [unwired: 1 out]
      n230 = Build Path(base path=w464, name or relative path="Data_get.cfg") -> (appended path=w466:path)
      n231 = call "SaveControlValues.vi"("file path"=w466, "vi path"=w463) -> ("error out"=w465:errorcluster)
      n232 = call <vilib>:"Simple Error Handler.vi"("error in (no error)"=w465) -> ()  [unwired: 4 in, 5 out]
    }
  }
